vi "DSF.Engine.Plugin.Shutdown.vi"(8 "error in (no error)":errorcluster, 11 "UDP Plugin in":refnum<class "DSF.Plugin.UDP.lvclass">) -> (0 "error out":errorcluster, 3 "UDP Plugin out":refnum<class "DSF.Plugin.UDP.lvclass">)   [LabVIEW 2017, in "DSF.Plugin.UDP.lvclass"]
uses:
  DSF.Plugin.UDP.lvclass
  Engine/Classes/Plugin/Plugin.lvclass
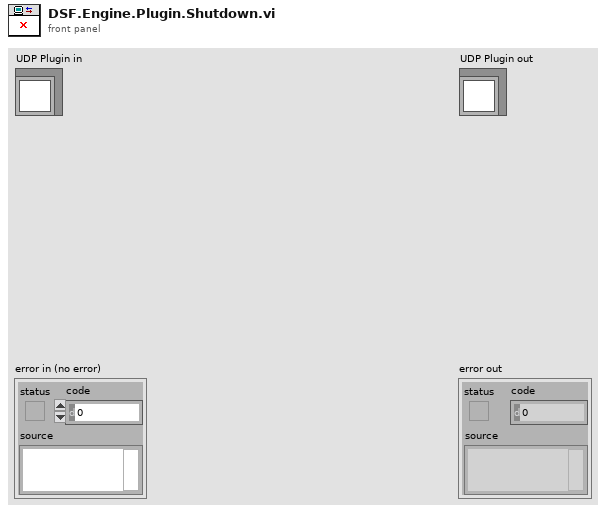
[diagram p1: front panel]
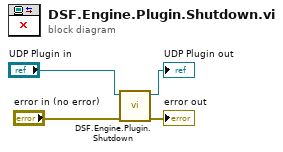
[diagram p0: block diagram]
diagram:
  n1 = call-parent "DSF.Engine.Plugin.Shutdown.vi"("error in (no error)"="error in (no error)", "Plugin in"="UDP Plugin in") -> ("error out"=→"error out":errorcluster, "Plugin out"=→"UDP Plugin out":refnum<class "DSF.Plugin.UDP.lvclass">)  [unwired: 8 in]
